vi "Ejemplo_FT.vi"() -> ()   [LabVIEW 2021]
panel:
  out "output array":dbl[](array[numeric])
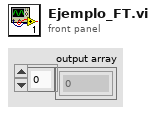
[diagram p1: front panel]
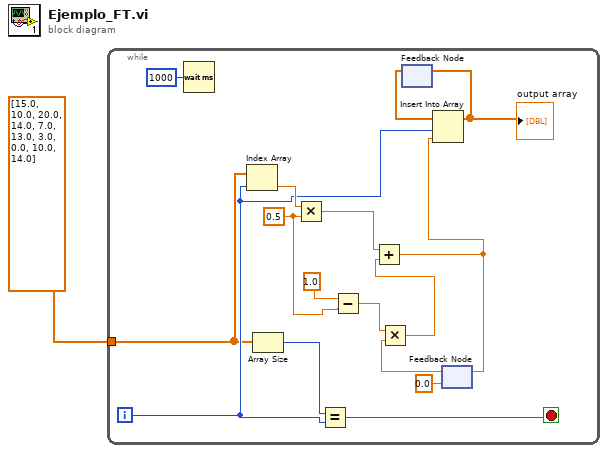
[diagram p0: block diagram]
diagram:
  n1 = while {
    tunnel: dbl[] [15.0, 10.0, 20.0, 14.0, 7.0, 13.0, 3.0, 0.0, 10.0, 14.0] -> [w4]
    i -> [w6]
    stop <- w8 stop-if-true
    w15 = 0.5 ("y")
    n2 = Wait (ms)(milliseconds to wait=u32 1000) -> ()  [unwired: 1 out]
    n3 = Index Array(array=w4, index=w6) -> (element=w10:dbl)
    n4 = Array Size(array=w4) -> (size(s)=w9:i32)
    n5 = Multiply(x=w10, y=w15) -> (x*y=w17:dbl)
    n6 = Equal?(x=w9, y=w6) -> (x = y?=w8:bool)
    n7 = Subtract(x=1.0, y=w15) -> (x-y=w14:dbl)
    n8 = feedback #1() -> (w3:dbl[])  [unwired: 1 in]
    n9 = feedback #2(0.0) -> (w12:dbl)
    n10 = Multiply(x=w14, y=w12) -> (x*y=w13:dbl)
    n11 = Add(x=w17, y=w13) -> (x+y=w5:dbl)
    n12 = Insert Into Array(array=w3, index=w6, new element=w5) -> (w2:dbl[])
    "output array" <- w2
    n13 = feedback-in #1(w2) -> ()
    n14 = feedback-in #2(w5) -> ()
  }
